vi "ZMC Close.vi"(8 "error in (no error)":errorcluster caption="错误输入（无错误）", 11 "handle":u32) -> (0 "error out":errorcluster caption="错误输出", 2 "function return":i32, 3 "handle out":u32)   [LabVIEW 2019, in "zauxdll.lvlib"]
doc: "int32 __stdcall ZMC_Close(ZMC_HANDLE handle);"
uses:
  zauxdll.lvlib
  zmotion.dll
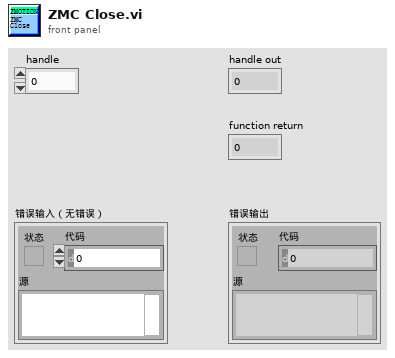
[diagram p1: front panel]
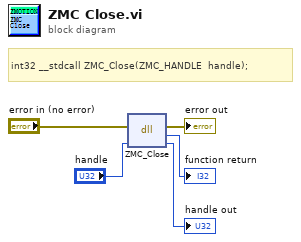
[diagram p0: block diagram]
diagram:
  # "int32 __stdcall ZMC_Close(ZMC_HANDLE  handle);"
  n1 = dll-call lib="C:/Users/VIC/Desktop/Standar Program/System/LLB/zmotion/zaux/zmotion.*" fn="ZMC_Close"(error in="error in (no error)", "handle"="handle") -> (error out=→"error out":errorcluster, "return type"=→"function return":i32, "handle"=→"handle out":u32)  [unwired: 2 in, 1 out]
